vi "(Old Driver) Block Write Multiple Iterator.vi"(8 "error in (no error)":errorcluster, 9 "Iterations (1000)":i32=1000, 10 "Channel Counts":i32[](array[numeric]), 11 "VMIC-5565":T1) -> (0 "error out":errorcluster, 1 "Histograms":T2(array[cluster]), 2 "Metrics":T3[](array[typedef]) {"Transfer Rate" format="%.2pB/s"; "Duration Std. Dev." format="%.0f µs"; "Duration Average" format="%.0f µs"}, 3 "VMIC-5565 out":T1)   [LabVIEW 2016]
uses:
  Controls/Throughput Metrics.ctl
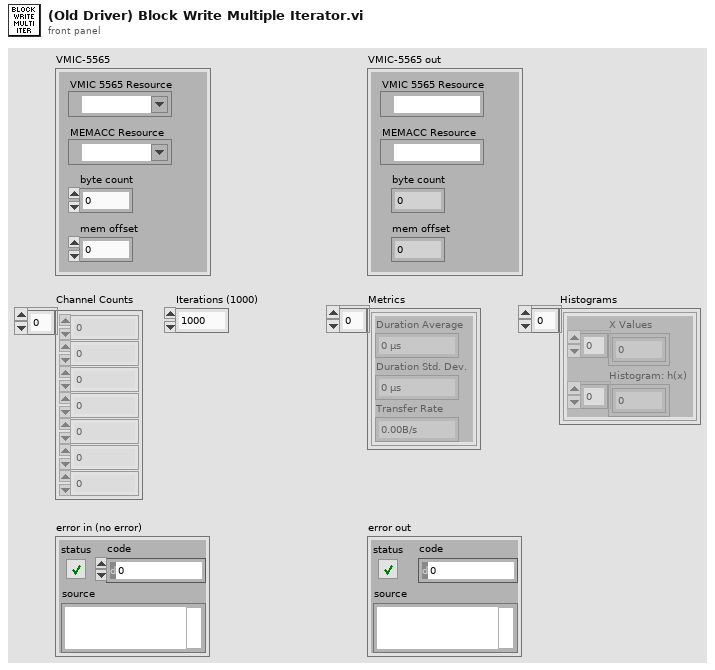
[diagram p1: front panel]
types:
  T1 = cluster{"VMIC 5565 Resource":refnum<visa-resource-name>, "MEMACC Resource":refnum<visa-resource-name>, "byte count":u32, "mem offset":u32}
  T2 = cluster{"X Values":dbl[], "Histogram: h(x)":i32[]}[]
  T3 = typedef "Throughput Metrics.ctl" = cluster{"Duration Average":u32, "Duration Std. Dev.":u32, "Transfer Rate":dbl}
  T4 = cluster{"X Values":dbl[], "Histogram: h(x)":i32[]}
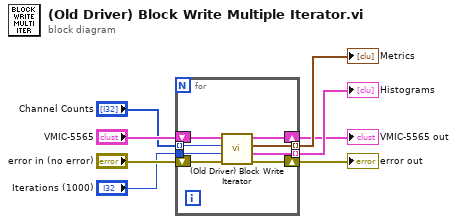
[diagram p0: block diagram]
diagram:
  n1 = for {
    shift-right: [w13] -> w5
    shift-left: "VMIC-5565" -> [w16]
    shift-right: [w14] -> w8
    shift-left: "error in (no error)" -> [w15]
    tunnel: "Channel Counts" -> [w12] mode=indexing
    tunnel: "Iterations (1000)" -> [w11]
    tunnel: [w10] -> w7 mode=indexing
    tunnel: [w9] -> w6 mode=indexing
    n2 = call "(Old Driver) Block Write Iterator.vi"("error in (no error)"=w15, "Iterations (1000)"=w11, "Channel Count"=w12, "VMIC-5565"=w16) -> ("error out"=w14:errorcluster, "Histogram Graph"=w9:T4, "Metrics"=w10:T3, "VMIC-5565 out"=w13:T1)  [unwired: 4 in]
  }
  "error out" <- w8
  "Metrics" <- w7
  "Histograms" <- w6
  "VMIC-5565 out" <- w5
